vi "RP ADC to Volts 1D.vi"(6 "osc_fpga_cnv_cnt_to_v method":bool, 7 "Max Volts":dbl=1.0, 11 "ADC data":i16[](array[numeric])) -> (3 "Volts":dbl[](array[numeric]))   [LabVIEW 2015]
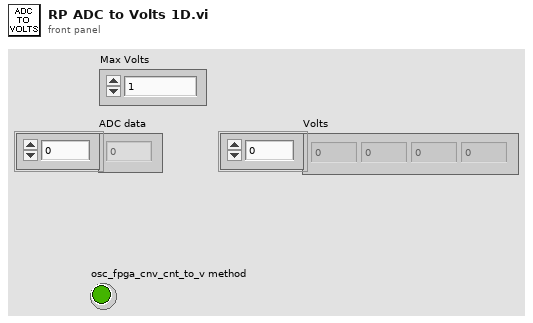
[diagram p1: front panel]
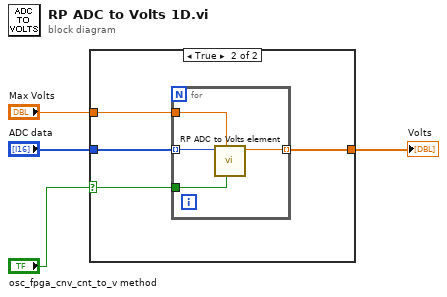
[diagram p0: block diagram]
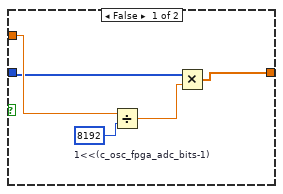
[diagram p2: hidden frame]
diagram:
  n1 = case shown="True" "osc_fpga_cnv_cnt_to_v method" {
    selector: "osc_fpga_cnv_cnt_to_v method" -> [_ w10]
    tunnel: "ADC data" -> [w6 w13]
    tunnel: [w5 w12] -> w3
    tunnel: "Max Volts" -> [w8 w11]
    frame False {
      w9 = 8192  # 1<<(c_osc_fpga_adc_bits-1)
      n2 = Divide(x=w8, y=w9) -> (x/y=w7:dbl)
      n3 = Multiply(x=w6, y=w7) -> (x*y=w5:dbl[])
    }
    frame True {
      n4 = for {
        tunnel: w13 -> [w17] mode=indexing
        tunnel: [w16] -> w12 mode=indexing
        tunnel: w10 -> [w15]
        tunnel: w11 -> [w14]
        n5 = call "RP ADC to Volts element.vi"("osc_fpga_cnv_cnt_to_v method"=w15, "Max Volts"=w14, "ADC data"=w17) -> ("Volts"=w16:dbl)  [unwired: 8 in]
      }
    }
  }
  "Volts" <- w3
